vi "Update Cursor.vi"(8 "error in (no error)":errorcluster, 10 "Tool Buttons":T1, 11 "UI Controller in":refnum<class "UI Controller.lvclass">) -> (0 "error out":errorcluster, 3 "UI Controller out":refnum<class "UI Controller.lvclass">)   [LabVIEW 2020, in "UI Controller.lvlib" / "UI Controller.lvclass"]
uses:
  UI Controller.lvclass
  Type Definitions/Tool Buttons.ctl
  UI Controller.lvclass/UI Controller.ctl
panel:
  # "NOTICE -- YOU MUST LEAVE THIS NOTICE IN PLACE.\n\nCopyright (c) 2017, LIANG LIU Shawn.Liu.cn@gmail.com\nAll rights reserved.\n\nRedistribution and use in source and binary forms, with or without modification, are permitted provided that the following conditions are met:\n-Redistributions of source code must retain the above copyright notice, this list of conditions and the following disclaimer.\n-Redistributions in binary form must reproduce the above copyright notice, this list of conditions and the following disclaimer in the documentation and/or other materials provided with the distribution.\n-Neither the name of the eLp nor the names of its contributors may be used to endorse or promote products derived from this software without specific prior written permission.\n\nTHIS SOFTWARE IS PROVIDED BY THE COPYRIGHT HOLDERS AND CONTRIBUTORS \"AS IS\" AND ANY EXPRESS OR IMPLIED WARRANTIES, INCLUDING, BUT NOT LIMITED TO, THE IMPLIED WARRANTIES OF MERCHANTABILITY AND FITNESS FOR A PARTICULAR PURPOSE ARE DISCLAIMED. IN NO EVENT SHALL THE COPYRIGHT HOLDER OR CONTRIBUTORS BE LIABLE FOR ANY DIRECT, INDIRECT, INCIDENTAL, SPECIAL, EXEMPLARY, OR CONSEQUENTIAL DAMAGES (INCLUDING, BUT NOT LIMITED TO, PROCUREMENT OF SUBSTITUTE GOODS OR SERVICES; LOSS OF USE, DATA, OR PROFITS; OR BUSINESS INTERRUPTION) HOWEVER CAUSED AND ON ANY THEORY OF LIABILITY, WHETHER IN CONTRACT, STRICT LIABILITY, OR TORT (INCLUDING NEGLIGENCE OR OTHERWISE) ARISING IN ANY WAY OUT OF THE USE OF THIS SOFTWARE, EVEN IF ADVISED OF THE POSSIBILITY OF SUCH DAMAGE."
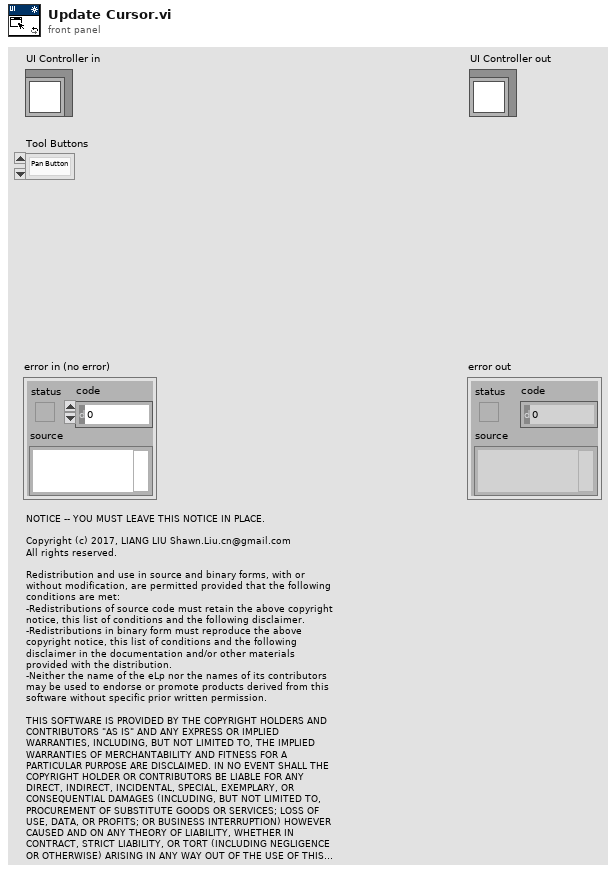
[diagram p1: front panel]
types:
  T1 = typedef "Tool Buttons.ctl" = enum32{"Pan Button", "Pencil Button", "Line Button", "Eraser Button", "Rectangle Select Button", "Deselect Button", "Crop Button", "Rotate Button", "Set Origin Button", "Zoom In Button", "Zoom Out Button"}
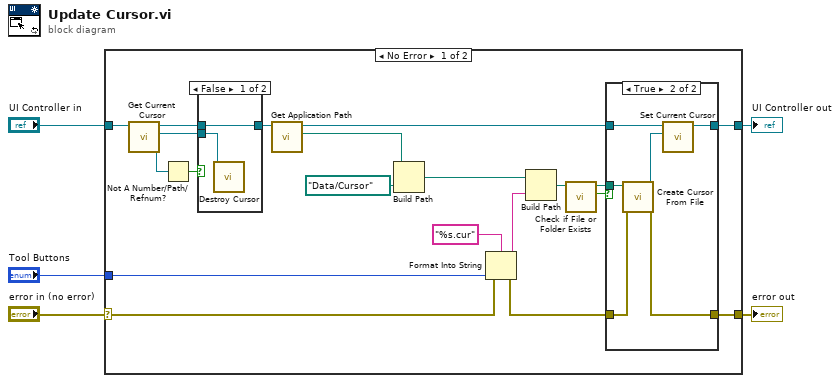
[diagram p0: block diagram]
diagram:
  n1 = case shown="No Error" "error in (no error)" {
    selector: "error in (no error)" -> [w21 w37]
    tunnel: "UI Controller in" -> [w24 w36]
    tunnel: [w23 w36] -> w4
    tunnel: "Tool Buttons" -> [w22 _]
    tunnel: [w7 w37] -> w1
    frame No Error {
      n2 = call "Get Current Cursor.vi"("UI Controller in"=w24) -> ("Current Cursor"=w12:refnum<k1>, "UI Controller out"=w11:refnum<class "UI Controller.lvclass">)  [unwired: 9 in]
      n3 = Not A Number/Path/Refnum?(number/path/refnum=w12) -> (NaN/Path/Refnum?=w13:bool)
      n4 = case shown="False" w13 {
        tunnel: w12 -> [w34 _]
        tunnel: w11 -> [w33 w35]
        tunnel: [w33 w35] -> w10
        frame False {
          n5 = call <vilib>:"Destroy Cursor.vi"("cursor ID"=w34) -> ()  [unwired: 9 in, 1 out]
        }
        frame True {
        }
      }
      n6 = call "Get Application Path.vi"("UI Controller in"=w10) -> ("Application Path"=w19:path, "UI Controller out"=w20:refnum<class "UI Controller.lvclass">)  [unwired: 9 in]
      n7 = Build Path(base path=w19, name or relative path=path "Data/Cursor") -> (appended path=w17:path)
      n8 = Format Into String(format string="%s.cur", error in=w21, w22) -> (resulting string=w14:string, error out=w6:errorcluster)  [unwired: 1 in]
      n9 = Build Path(base path=w17, name or relative path=w14) -> (appended path=w15:path)
      n10 = call <vilib>:"Check if File or Folder Exists.vi"("path"=w15) -> ("file or folder exists?"=w8:bool, "dup path"=w9:path)  [unwired: 8 in, 1 out]
      n11 = case shown="True" w8 {
        tunnel: [w26 w32] -> w23
        tunnel: w20 -> [w26 w31]
        tunnel: w9 -> [_ w30]
        tunnel: [w25 w28] -> w7
        tunnel: w6 -> [w25 w27]
        frame False {
        }
        frame True {
          n12 = call <vilib>:"Create Cursor From File.vi"("error in (no error)"=w27, "cursor file"=w30) -> ("error out"=w28:errorcluster, "cursor ID"=w29:refnum<k1>)  [unwired: 8 in]
          n13 = call "Set Current Cursor.vi"("Current Cursor"=w29, "UI Controller in"=w31) -> ("UI Controller out"=w32:refnum<class "UI Controller.lvclass">)  [unwired: 9 in]
        }
      }
    }
    frame Error {
    }
  }
  "error out" <- w1
  "UI Controller out" <- w4
